vi "Select_SglVar.vi"(8 "error in (no error)":errorcluster, 10 "varName":string, 11 "mupExpr in":refnum<data-value>) -> (0 "error out":errorcluster, 3 "mupExpr out":refnum<data-value>)   [LabVIEW 2015, in "mupExpr.lvclass"]
doc: "Select the variable, by name, for use in single variable evaluation.\nReturns error if the input variable is not found."
uses:
  mupExpr.lvclass
  mupExpr.lvclass/mupExpr.ctl
panel:
  # "Select the variable, by name, for use in single variable evaluation.\nReturns error if the input variable is not found."
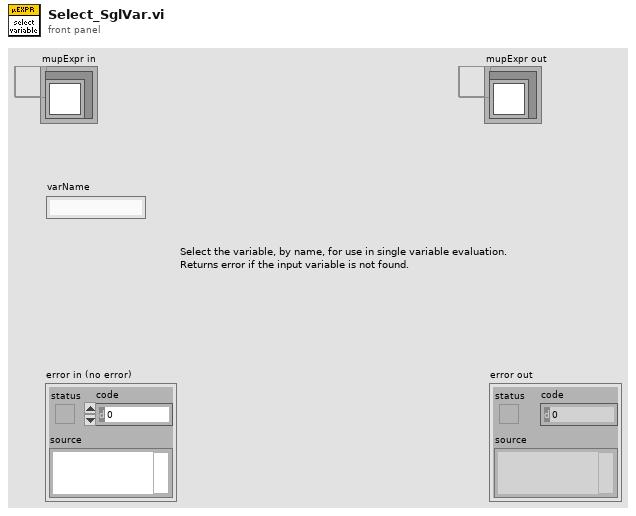
[diagram p1: front panel]
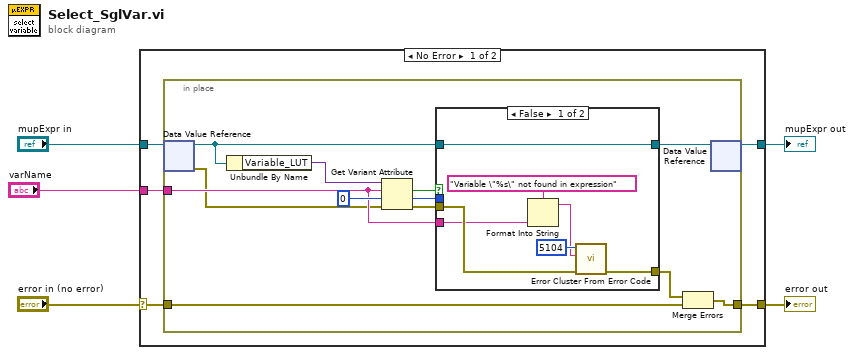
[diagram p0: block diagram]
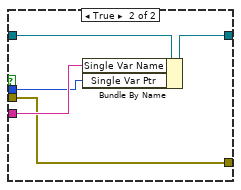
[diagram p2: hidden frame]
diagram:
  n1 = case shown="No Error" "error in (no error)" {
    selector: "error in (no error)" -> [w10 w36]
    tunnel: [w8 w36] -> w4
    tunnel: [w6 w35] -> w2
    tunnel: "mupExpr in" -> [w7 w35]
    tunnel: "varName" -> [w9 _]
    frame No Error {
      n2 = in-place {
        in-place-border: w10 -> [w12]
        in-place-border: w9 -> [w18]
        in-place-border: [w11] -> w8
        n3 = in-place-dvr #1(w7) -> (w16:refnum<class "mupExpr.lvclass">, w14:errorcluster)
        n4 = Unbundle By Name(w16) -> ("Variable_LUT"=w22:variant)
        n5 = Get Variant Attribute(Variant=w22, name=w18, default value (empty Variant)=u64 0, error in=w14) -> (found=w21:bool, value=w19:u64, error out=w17:errorcluster)  [unwired: 1 out]
        n6 = case shown="False" w21 {
          tunnel: w19 -> [_ w32]
          tunnel: w16 -> [w29 w34]
          tunnel: w18 -> [w25 w33]
          tunnel: [w29 w31] -> w15
          tunnel: w17 -> [w28 w30]
          tunnel: [w23 w30] -> w13
          frame False {
            n7 = Format Into String(format string="Variable \"%s\" not found in expression" ("error message (\"\")"), w25) -> (resulting string=w24:string)  [unwired: 2 in, 1 out]
            n8 = call <vilib>:"Error Cluster From Error Code.vi"("error in (no error)"=w28, "error message (\"\")"=w24, "error code (0)"=5104) -> ("error out"=w23:errorcluster)  [unwired: 6 in]
          }
          frame True {
            n9 = Bundle By Name(cluster=w34, "Single Var Name"=w33, "Single Var Ptr"=w32) -> (w31:refnum<class "mupExpr.lvclass">)
          }
        }
        n10 = Merge Errors(w13, w12) -> (w11:errorcluster)
        n11 = in-place-dvr #1(w15) -> (w6:refnum<data-value>)  [unwired: 1 out]
      }
    }
    frame Error {
    }
  }
  "error out" <- w4
  "mupExpr out" <- w2
